vi "FVT.vi"(7 "FrequencyCounter":refnum<visa-resource-name>, 8 "error in":errorcluster, 9 "connection information":path, 10 "System Number":string, 11 "Arduino":refnum<visa-resource-name>) -> (0 "error out":errorcluster, 3 "Arduino out":refnum<visa-resource-name>)   [LabVIEW 2024]
uses:
  <vilib>/addons/database/Connection.llb/DB Tools Open Connec (Path).vi
  Agilent 532XX Series/Public/Configure/Measurement/Configure Measurement (Frequency).vi
  <vilib>/Utility/file.llb/Write Delimited Spreadsheet (string).vi
  <vilib>/addons/database/_DB Variant To Data/Database Variant To Data.xnode
  <vilib>/addons/database/NI_Database_API.lvlib
  Agilent 532XX Series/Agilent 532XX Series.lvlib
panel:
  out "OscVoltage":string
  out "TimeStart":string
  out "StartTime":string
  out "FirstPrint":bool
  out "FirstTime":bool
  out "Path":string
  out "PDF Path":string
  out "Work Order":string
  out "Unit_Number":string
  out "Serial Numbers":string[](array[string])
  in  "System Status":string
  out "Frequency":string
  out "Temperature":string
  out "Nominal Frequency":string
  in  "DC_SN":string
  out "IsSine":bool=TRUE
types:
  T1 = typedef "NI_Database_API.lvlib/Conn ObjectReference.ctl" = refnum<k1>
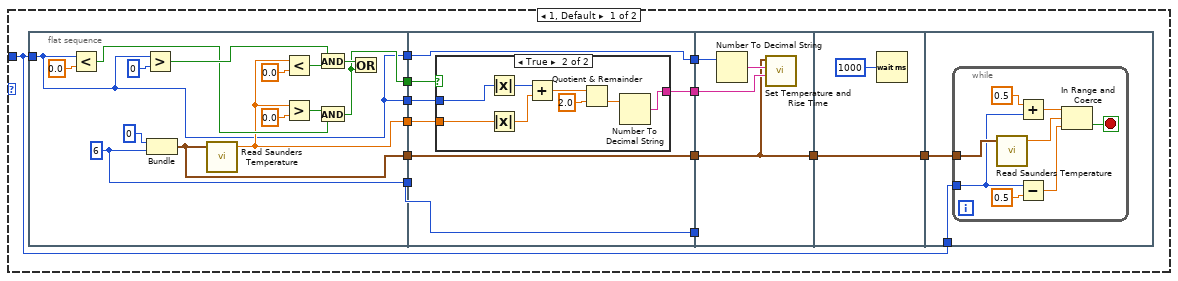
[diagram p2: hidden frame]
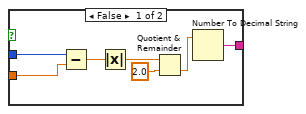
[diagram p3: hidden frame]
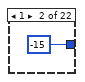
[diagram p4: hidden frame]
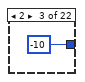
[diagram p5: hidden frame]
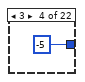
[diagram p6: hidden frame]
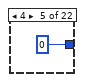
[diagram p7: hidden frame]
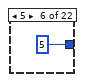
[diagram p8: hidden frame]
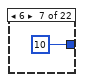
[diagram p9: hidden frame]
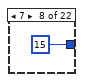
[diagram p10: hidden frame]
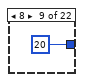
[diagram p11: hidden frame]
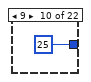
[diagram p12: hidden frame]
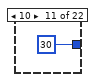
[diagram p13: hidden frame]
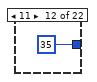
[diagram p14: hidden frame]
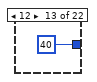
[diagram p15: hidden frame]
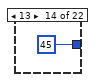
[diagram p16: hidden frame]
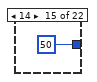
[diagram p17: hidden frame]
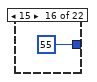
[diagram p18: hidden frame]
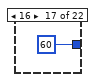
[diagram p19: hidden frame]
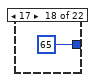
[diagram p20: hidden frame]
diagram:
  n1 = flat-sequence {
    tunnel: "Arduino" -> [w19]
    tunnel: "error in" -> [w18]
    tunnel: [w17] -> w2
    tunnel: [w16] -> w1
    tunnel: [w34] -> w6
    tunnel: [w35] -> w4
    tunnel: w2 -> [w37]
    tunnel: w1 -> [w36]
    tunnel: w6 -> [w733]
    tunnel: [w733] -> w5
    tunnel: w4 -> [w732]
    tunnel: [w732] -> w3
    tunnel: [w773] -> w11
    tunnel: w5 -> [w773]
    tunnel: [w772] -> w9
    tunnel: w3 -> [w772]
    tunnel: [w771] -> w7
    tunnel: w11 -> [w779]
    tunnel: [w779] -> w10
    tunnel: w9 -> [w778]
    tunnel: [w778] -> w8
    tunnel: w7 -> [w777]
    tunnel: w10 -> [w785]
    tunnel: w8 -> [w784]
    tunnel: [w785] -> w13
    tunnel: [w784] -> w12
    frame #0 {
      n2 = Build Array("<48,0>" ("string"), "<50,0>" ("string"), "<52,0>" ("string")) -> (w20:string[])
      n3 = Get Date/Time In Seconds() -> (seconds since 1Jan1904=w29:timestamp)
      n4 = Format Date/Time String(time format string (%c)="%x_%I-%M" ("string"), seconds (now)=w29) -> (date/time string=w28:string)  [unwired: 1 in]
      n5 = call "Arduino Command Builder.vi"("error in"=w18, "Commands"=w20, "Arduino in"=w19) -> ("error out"=w17:errorcluster, "Arduino out"=w16:refnum<visa-resource-name>)  [unwired: 7 in]
      n6 = Search and Replace String(replace all?=TRUE ("replace all? (F)"), input string=w28, search string="/", replace string="-" ("replace string (\"\")")) -> (result string=→"StartTime":string)  [unwired: 4 in, 3 out]
      "FirstTime" <- TRUE ("FirstTime")
      "FirstPrint" <- TRUE ("FirstPrint")
      "Serial Numbers" <- string[] []
    }
    frame #1 {
      n7 = for {
        N: 22 -> [_]
        shift-right: [w40] -> w34
        shift-left: w37 -> [w43]
        shift-right: [w41] -> w35
        shift-left: w36 -> [w42]
        i -> [w39]
        n8 = flat-sequence {
          tunnel: w39 -> [w44]
          tunnel: w43 -> [w156]
          tunnel: w42 -> [w155]
          tunnel: [w154] -> w40
          tunnel: [w153] -> w41
          tunnel: w39 -> [w152]
          frame #0 {
            n9 = case shown="0, Default" w44 {
              tunnel: [-20 -15 -10 -5 0 5 10 15 20 25 30 35 40 45 50 55 60 65 70 75 80 85] -> w45
              frame 0, Default {
              }
              frame 1 {
              }
              frame 2 {
              }
              frame 3 {
              }
              frame 4 {
              }
              frame 5 {
              }
              frame 6 {
              }
              frame 7 {
              }
              frame 8 {
              }
              frame 9 {
              }
              frame 10 {
              }
              frame 11 {
              }
              frame 12 {
              }
              frame 13 {
              }
              frame 14 {
              }
              frame 15 {
              }
              frame 16 {
              }
              frame 17 {
              }
              frame 18 {
              }
              frame 19 {
              }
              frame 20 {
              }
              frame 21 {
              }
            }
            n10 = case shown="0" w44 {
              tunnel: w45 -> [w46 w112]
              frame 1, Default {
                n11 = flat-sequence {
                  tunnel: w46 -> [w59]
                  tunnel: [w59] -> w58
                  tunnel: [w73] -> w57
                  tunnel: [w71] -> w56
                  tunnel: [w61] -> w55
                  tunnel: [w60] -> w54
                  tunnel: [w59] -> w53
                  tunnel: w58 -> [w80]
                  tunnel: [w80] -> w52
                  tunnel: [w74] -> w51
                  tunnel: w57 -> [w79]
                  tunnel: [w79] -> w50
                  tunnel: w56 -> [w78]
                  tunnel: [w78] -> w49
                  tunnel: w55 -> [w77]
                  tunnel: w54 -> [w76]
                  tunnel: w53 -> [w75]
                  tunnel: [w96] -> w48
                  tunnel: w52 -> [w98]
                  tunnel: w51 -> [w97]
                  tunnel: w50 -> [_]
                  tunnel: w49 -> [w96]
                  tunnel: [w100] -> w47
                  tunnel: w48 -> [w100]
                  tunnel: w46 -> [w103]
                  tunnel: w47 -> [w102]
                  frame #0 {
                    w73 = 6
                    n12 = Less?(x=w59, y=0.0) -> (x < y?=w65:bool)
                    n13 = Greater?(x=w59, y=0) -> (0:w68:bool)
                    n14 = Bundle(0, w73) -> (w71:cluster{i32, i32})  [unwired: 1 in]
                    n15 = call "Read Saunders Temperature.vi"("Device"=w71) -> ("Temperature"=w60:dbl)  [unwired: 3 in, 1 out]
                    n16 = Less?(x=w60, y=0.0) -> (x < y?=w67:bool)
                    n17 = Greater?(x=w60, y=0.0) -> (0:w66:bool)
                    n18 = And(x=w68, y=w67) -> (x .and. y?=w64:bool)
                    n19 = And(x=w66, y=w65) -> (x .and. y?=w61:bool)
                    n20 = Or(x=w64, y=w61) -> ()  [unwired: 1 out]
                  }
                  frame #1 {
                    n21 = case shown="True" w77 {
                      tunnel: w76 -> [w86 w94]
                      tunnel: w75 -> [w87 w95]
                      tunnel: [w82 w91] -> w74
                      frame False {
                        n22 = Subtract(x=w87, y=w86) -> (x-y=w85:dbl)
                        n23 = Absolute Value(x=w85) -> (abs(x)=w81:dbl)
                        n24 = Quotient & Remainder(x=w81, y=2.0) -> (floor(x/y)=w83:dbl)  [unwired: 1 out]
                        n25 = Number To Decimal String(number=w83) -> (decimal integer string=w82:string)  [unwired: 1 in]
                      }
                      frame True {
                        n26 = Absolute Value(x=w95) -> (abs(x)=w92:i32)
                        n27 = Absolute Value(x=w94) -> (abs(x)=w93:dbl)
                        n28 = Add(x=w92, y=w93) -> (x+y=w88:dbl)
                        n29 = Quotient & Remainder(x=w88, y=2.0) -> (floor(x/y)=w89:dbl)  [unwired: 1 out]
                        n30 = Number To Decimal String(number=w89) -> (decimal integer string=w91:string)  [unwired: 1 in]
                      }
                    }
                  }
                  frame #2 {
                    n31 = Number To Decimal String(number=w98) -> (decimal integer string=w99:string)  [unwired: 1 in]
                    n32 = call "Set Temperature and Rise Time.vi"("Slew Time String"=w97, "Temperature String"=w99, "Device"=w96) -> ()  [unwired: 3 in, 1 out]
                  }
                  frame #3 {
                    n33 = Wait (ms)(milliseconds to wait=u32 1000) -> ()  [unwired: 1 out]
                  }
                  frame #4 {
                    n34 = while {
                      tunnel: w102 -> [w111]
                      tunnel: w103 -> [w108]
                      stop <- w110 stop-if-true
                      n35 = call "Read Saunders Temperature.vi"("Device"=w111) -> ("Temperature"=w109:dbl)  [unwired: 3 in, 1 out]
                      n36 = Add(x=0.5, y=w108) -> (x+y=w104:dbl)
                      n37 = Subtract(x=w108, y=0.5) -> (x-y=w106:dbl)
                      n38 = In Range and Coerce(upper limit=w104, x=w109, lower limit=w106) -> (In Range?=w110:bool)  [unwired: 1 out]
                    }
                  }
                }
              }
              frame 0 {
                n39 = flat-sequence {
                  tunnel: w112 -> [w117]
                  frame #0 {
                    n40 = Number To Decimal String(number=w117) -> (decimal integer string=w119:string)  [unwired: 1 in]
                    n41 = Bundle(0, 6) -> (w113:cluster{i32, i32})  [unwired: 1 in]
                    n42 = Wait (ms)(milliseconds to wait=u32 1000) -> ()  [unwired: 1 out]
                    n43 = while {
                      tunnel: w113 -> [w127]
                      tunnel: w117 -> [w124]
                      stop <- w126 stop-if-true
                      n44 = call "Read Saunders Temperature.vi"("Device"=w127) -> ("Temperature"=w125:dbl)  [unwired: 3 in, 1 out]
                      n45 = Add(x=0.5, y=w124) -> (x+y=w120:dbl)
                      n46 = Subtract(x=w124, y=0.5) -> (x-y=w122:dbl)
                      n47 = In Range and Coerce(upper limit=w120, x=w125, lower limit=w122) -> (In Range?=w126:bool)  [unwired: 1 out]
                    }
                    n48 = call "Set Temperature and Rise Time.vi"("Slew Time String"="0", "Temperature String"=w119, "Device"=w113) -> ()  [unwired: 3 in, 1 out]
                  }
                  frame #1 {
                    n49 = Wait (ms)(milliseconds to wait=u32 600000) -> ()  [unwired: 1 out]
                  }
                }
              }
            }
          }
          frame #1 {
            n50 = Wait (ms)(milliseconds to wait=u32 60000) -> ()  [unwired: 1 out]
          }
          frame #2 {
            n51 = for {
              N: 32 -> [_]
              shift-right: [w161] -> w154
              shift-left: w156 -> [w163]
              shift-right: [w160] -> w153
              shift-left: w155 -> [w162]
              tunnel: w152 -> [w158]
              i -> [w159]
              n52 = for {
                N: 8 -> [_]
                shift-right: [w172] -> w161
                shift-left: w163 -> [w177]
                shift-right: [w167] -> w160
                shift-left: w162 -> [w176]
                tunnel: w159 -> [w175]
                tunnel: w158 -> [w166]
                i -> [w178]
                n53 = flat-sequence {
                  tunnel: w177 -> [w181]
                  tunnel: w176 -> [w180]
                  tunnel: [w179] -> w171
                  tunnel: [w180] -> w168
                  tunnel: w178 -> [w185]
                  tunnel: w175 -> [w183]
                  tunnel: [w182] -> w174
                  tunnel: [w217] -> w173
                  tunnel: w171 -> [w216]
                  tunnel: [w216] -> w170
                  tunnel: [w215] -> w169
                  tunnel: w168 -> [w215]
                  tunnel: [w184] -> w165
                  tunnel: w174 -> [w270]
                  tunnel: w173 -> [w269]
                  tunnel: [w268] -> w172
                  tunnel: w170 -> [w267]
                  tunnel: w169 -> [w266]
                  tunnel: [w265] -> w167
                  tunnel: w166 -> [w264]
                  tunnel: w165 -> [w263]
                  frame #0 {
                    n54 = call <vilib>:"Clear Errors.vi"("error in (no error)"=w181) -> ("error out"=w179:errorcluster)  [unwired: 5 in, 1 out]
                  }
                  frame #1 {
                    n55 = local write "DC_SN"("" ("DC.SN")) -> ()
                    n56 = local read "System Number"() -> (w203:string)
                    n57 = local read "connection information"() -> (w186:path)
                    n58 = Increment(x=w185) -> (x+1=w202:i32)
                    n59 = Number To Decimal String(number=w202) -> (decimal integer string=w204:string)  [unwired: 1 in]
                    n60 = Concatenate Strings("WHERE System=" ("SQL Query"), w203, " AND Rack=", w204, ";" ("string")) -> (w187:string)
                    n61 = call-poly <vilib>:"DB Tools Open Connection.vi"("connection information"=w186) -> ("error out"=w197:errorcluster, "connection reference"=w198:T1)  [unwired: 7 in]
                    n62 = call <vilib>:"DB Tools Select Data.vi"("condition"=w187, "error in (no error)"=w197, "columns"=string[] ["Position"], "table"="ACTIVE", "connection reference"=w198) -> ("error out"=w194:errorcluster, "data"=w192:variant[][], "connection reference out"=w196:T1)  [unwired: 1 in]
                    n63 = xnode "Database Variant To Data"("database variant"=w192, "error in (no error)"=w194, "type"=string[][] [] ("DC.SN")) -> ("data"=w191:string[][], "error out"=w195:errorcluster)
                    n64 = call <vilib>:"DB Tools Close Connection.vi"("error in (no error)"=w195, "connection reference"=w196) -> ("error out"=w188:errorcluster)  [unwired: 5 in]
                    n65 = Index Array(array=w191, index (row)=0 ("disabled index (row)"), index (col)=0 ("disabled index (col)")) -> (element=w214:string)
                    n66 = Unbundle By Name(w188) -> ("status"=w201:bool)
                    n67 = call <vilib>:"Delimited String to 1D String Array.vi"("delimiter"=",", "delimited string"=w214) -> ("string array"=w211:string[])  [unwired: 9 in]
                    n68 = Not(x=w201) -> (.not. x?=w200:bool)
                    n69 = Index Array(array=w211, index=w183) -> (element=w210:string)
                    n70 = Increment(x=w183) -> (x+1=w217:i32)
                    n71 = Equal?(x="1", y=w210) -> (x = y?=w199:bool)
                    n72 = Increment(x=w185) -> (x+1=w182:i32)
                    n73 = And(x=w199, y=w200) -> (x .and. y?=w184:bool)
                  }
                  frame #2 {
                    n74 = case shown="True" w263 {
                      tunnel: w270 -> [_ w307]
                      tunnel: w269 -> [_ w306]
                      tunnel: [w271 w302] -> w268
                      tunnel: w267 -> [w271 w305]
                      tunnel: w266 -> [w272 w304]
                      tunnel: [w272 w301] -> w265
                      tunnel: w264 -> [_ w294]
                      frame False {
                      }
                      frame True {
                        n75 = flat-sequence {
                          tunnel: w306 -> [w309]
                          tunnel: w307 -> [w308]
                          tunnel: [w308] -> w278
                          tunnel: [w309] -> w277
                          tunnel: [w310] -> w276
                          tunnel: [w505] -> w286
                          tunnel: w278 -> [w509]
                          tunnel: w277 -> [w508]
                          tunnel: w276 -> [w510]
                          tunnel: [w510] -> w275
                          tunnel: [w507] -> w274
                          tunnel: [w506] -> w273
                          tunnel: [w596] -> w302
                          tunnel: w305 -> [w598]
                          tunnel: w304 -> [w599]
                          tunnel: [w597] -> w301
                          tunnel: [w592] -> w295
                          tunnel: [w595] -> w287
                          tunnel: w286 -> [w595]
                          tunnel: [w594] -> w279
                          tunnel: w275 -> [w593]
                          tunnel: w274 -> [w592]
                          tunnel: w273 -> [w594]
                          tunnel: [w609] -> w296
                          tunnel: w295 -> [w609]
                          tunnel: [w608] -> w288
                          tunnel: w287 -> [w608]
                          tunnel: [w607] -> w280
                          tunnel: w279 -> [w607]
                          tunnel: [w620] -> w300
                          tunnel: [w613] -> w297
                          tunnel: w296 -> [w613]
                          tunnel: [w612] -> w289
                          tunnel: w288 -> [w612]
                          tunnel: [w611] -> w281
                          tunnel: w280 -> [w611]
                          tunnel: [w624] -> w303
                          tunnel: [w623] -> w298
                          tunnel: [w622] -> w290
                          tunnel: [w621] -> w282
                          tunnel: w281 -> [w621]
                          tunnel: w289 -> [w622]
                          tunnel: w297 -> [w623]
                          tunnel: w300 -> [w624]
                          tunnel: w303 -> [w626]
                          tunnel: [w630] -> w299
                          tunnel: w298 -> [w630]
                          tunnel: [w629] -> w291
                          tunnel: w290 -> [w629]
                          tunnel: [w628] -> w283
                          tunnel: w282 -> [w628]
                          tunnel: w299 -> [w654]
                          tunnel: [w653] -> w292
                          tunnel: w291 -> [w653]
                          tunnel: [w652] -> w284
                          tunnel: w283 -> [w652]
                          tunnel: w294 -> [w661]
                          tunnel: [w660] -> w293
                          tunnel: w292 -> [w660]
                          tunnel: [w659] -> w285
                          tunnel: w284 -> [w659]
                          tunnel: w293 -> [w722]
                          tunnel: w285 -> [w721]
                          frame #0 {
                            n76 = case shown="2" w308 {
                              tunnel: ["<42,0>" ("string") "<42,1>" ("string") "<42,0>" ("string") "<42,1>" ("string") "<42,0>" ("string") "<42,1>" ("string") "<42,0>" ("string") "<42,1>" ("string")] -> w316
                              tunnel: ["<44,0>" ("string") "<44,0>" ("string") "<44,1>" ("string") "<44,1>" ("string") "<44,0>" ("string") "<44,0>" ("string") "<44,1>" ("string") "<44,1>" ("string")] -> w317
                              tunnel: ["<46,0>" ("string") "<46,0>" ("string") "<46,0>" ("string") "<46,0>" ("string") "<46,1>" ("string") "<46,1>" ("string") "<46,1>" ("string") "<46,1>" ("string")] -> w318
                              frame 1, Default {
                              }
                              frame 2 {
                              }
                              frame 3 {
                              }
                              frame 4 {
                              }
                              frame 5 {
                              }
                              frame 6 {
                              }
                              frame 7 {
                              }
                              frame 8 {
                              }
                            }
                            n77 = case shown="2" w309 {
                              tunnel: ["<32,0>" ("string") "<32,0>" ("string") "<32,0>" ("string") "<32,0>" ("string") "<32,0>" ("string") "<32,0>" ("string") "<32,0>" ("string") "<32,0>" ("string") "<32,0>" ("string") "<32,0>" ("string") "<32,0>" ("string") "<32,0>" ("string") "<32,0>" ("string") "<32,0>" ("string") "<32,0>" ("string") "<32,0>" ("string") "<32,1>" ("string") "<32,1>" ("string") "<32,1>" ("string") "<32,1>" ("string") "<32,1>" ("string") "<32,1>" ("string") "<32,1>" ("string") "<32,1>" ("string") "<32,1>" ("string") "<32,1>" ("string") "<32,1>" ("string") "<32,1>" ("string") "<32,1>" ("string") "<32,1>" ("string") "<32,1>" ("string") "<32,1>" ("string")] -> w315
                              tunnel: ["<30,0>" ("string") "<30,0>" ("string") "<30,0>" ("string") "<30,0>" ("string") "<30,0>" ("string") "<30,0>" ("string") "<30,0>" ("string") "<30,0>" ("string") "<30,1>" ("string") "<30,1>" ("string") "<30,1>" ("string") "<30,1>" ("string") "<30,1>" ("string") "<30,1>" ("string") "<30,1>" ("string") "<30,1>" ("string") "<30,0>" ("string") "<30,0>" ("string") "<30,0>" ("string") "<30,0>" ("string") "<30,0>" ("string") "<30,0>" ("string") "<30,0>" ("string") "<30,0>" ("string") "<30,1>" ("string") "<30,1>" ("string") "<30,1>" ("string") "<30,1>" ("string") "<30,1>" ("string") "<30,1>" ("string") "<30,1>" ("string") "<30,1>" ("string")] -> w314
                              tunnel: ["<28,0>" ("string") "<28,0>" ("string") "<28,0>" ("string") "<28,0>" ("string") "<28,1>" ("string") "<28,1>" ("string") "<28,1>" ("string") "<28,1>" ("string") "<28,0>" ("string") "<28,0>" ("string") "<28,0>" ("string") "<28,0>" ("string") "<28,1>" ("string") "<28,1>" ("string") "<28,1>" ("string") "<28,1>" ("string") "<28,0>" ("string") "<28,0>" ("string") "<28,0>" ("string") "<28,0>" ("string") "<28,1>" ("string") "<28,1>" ("string") "<28,1>" ("string") "<28,1>" ("string") "<28,0>" ("string") "<28,0>" ("string") "<28,0>" ("string") "<28,0>" ("string") "<28,1>" ("string") "<28,1>" ("string") "<28,1>" ("string") "<28,1>" ("string")] -> w313
                              tunnel: ["<26,0>" ("string") "<26,0>" ("string") "<26,1>" ("string") "<26,1>" ("string") "<26,0>" ("string") "<26,0>" ("string") "<26,1>" ("string") "<26,1>" ("string") "<26,0>" ("string") "<26,0>" ("string") "<26,1>" ("string") "<26,1>" ("string") "<26,0>" ("string") "<26,0>" ("string") "<26,1>" ("string") "<26,1>" ("string") "<26,0>" ("string") "<26,0>" ("string") "<26,1>" ("string") "<26,1>" ("string") "<26,0>" ("string") "<26,0>" ("string") "<26,1>" ("string") "<26,1>" ("string") "<26,0>" ("string") "<26,0>" ("string") "<26,1>" ("string") "<26,1>" ("string") "<26,0>" ("string") "<26,0>" ("string") "<26,1>" ("string") "<26,1>" ("string")] -> w312
                              tunnel: ["<24,0>" ("string") "<24,1>" ("string") "<24,0>" ("string") "<24,1>" ("string") "<24,0>" ("string") "<24,1>" ("string") "<24,0>" ("string") "<24,1>" ("string") "<24,0>" ("string") "<24,1>" ("string") "<24,0>" ("string") "<24,1>" ("string") "<24,0>" ("string") "<24,1>" ("string") "<24,0>" ("string") "<24,1>" ("string") "<24,0>" ("string") "<24,1>" ("string") "<24,0>" ("string") "<24,1>" ("string") "<24,0>" ("string") "<24,1>" ("string") "<24,0>" ("string") "<24,1>" ("string") "<24,0>" ("string") "<24,1>" ("string") "<24,0>" ("string") "<24,1>" ("string") "<24,0>" ("string") "<24,1>" ("string") "<24,0>" ("string") "<24,1>" ("string")] -> w311
                              frame 1, Default {
                              }
                              frame 2 {
                              }
                              frame 3 {
                              }
                              frame 4 {
                              }
                              frame 5 {
                              }
                              frame 6 {
                              }
                              frame 7 {
                              }
                              frame 8 {
                              }
                              frame 9 {
                              }
                              frame 10 {
                              }
                              frame 11 {
                              }
                              frame 12 {
                              }
                              frame 13 {
                              }
                              frame 14 {
                              }
                              frame 15 {
                              }
                              frame 16 {
                              }
                              frame 17 {
                              }
                              frame 18 {
                              }
                              frame 19 {
                              }
                              frame 20 {
                              }
                              frame 21 {
                              }
                              frame 22 {
                              }
                              frame 23 {
                              }
                              frame 24 {
                              }
                              frame 25 {
                              }
                              frame 26 {
                              }
                              frame 27 {
                              }
                              frame 28 {
                              }
                              frame 29 {
                              }
                              frame 30 {
                              }
                              frame 31 {
                              }
                              frame 32 {
                              }
                            }
                            n78 = Build Array(w316, w317, w318, w311, w312, w313, w314, w315) -> (w310:string[])
                          }
                          frame #1 {
                            # "Gets the latest TimeStart from this System/Rack/Position meaning it will be associated with the oscillator that is currently in the spot"
                            n79 = local read "connection information"() -> (w514:path)
                            n80 = local read "System Number"() -> (w547:string)
                            n81 = Number To Decimal String(number=w509) -> (decimal integer string=w505:string)  [unwired: 1 in]
                            n82 = Number To Decimal String(number=w508) -> (decimal integer string=w506:string)  [unwired: 1 in]
                            n83 = Concatenate Strings("WHERE SystemNumber=" ("SQL Query"), w547, "AND RackNumber=" ("string"), w505, "AND PositionNumber=" ("string"), w506, "ORDER BY TimeStart DESC" ("string")) -> (w513:string)
                            n84 = call-poly <vilib>:"DB Tools Open Connection.vi"("connection information"=w514) -> ("error out"=w521:errorcluster, "connection reference"=w522:T1)  [unwired: 7 in]
                            n85 = call <vilib>:"DB Tools Select Data.vi"("condition"=w513, "error in (no error)"=w521, "table"="MASTER", "connection reference"=w522) -> ("error out"=w518:errorcluster, "data"=w516:variant[][], "connection reference out"=w520:T1)  [unwired: 2 in]
                            n86 = xnode "Database Variant To Data"("database variant"=w516, "error in (no error)"=w518, "type"=string[][] [] ("DC.SN")) -> ("data"=w512:string[][], "error out"=w519:errorcluster)
                            n87 = call <vilib>:"DB Tools Close Connection.vi"("error in (no error)"=w519, "connection reference"=w520) -> ("error out"=w511:errorcluster)  [unwired: 5 in]
                            n88 = Index Array(array=w512, index (row)=0 ("disabled index (row)")) -> (element=w526:string[])  [unwired: 1 in]
                            n89 = Unbundle By Name(w511) -> ("status"=w532:bool)
                            n90 = Index Array(array=w526, index=9) -> (element=→"OscVoltage":string)
                            n91 = Index Array(array=w526, index=1) -> (element=w525:string)
                            n92 = Index Array(array=w526, index=2) -> (element=w523:string)
                            n93 = Index Array(array=w526, index=7) -> (element=→"TimeStart":string)
                            n94 = Index Array(array=w526, index=8) -> (element=w540:string)
                            n95 = Index Array(array=w526, index=0) -> (element=w539:string)
                            n96 = Index Array(array=w526, index=12) -> (element=w504:string)
                            n97 = Index Array(array=w526, index=10) -> (element=w541:string)
                            n98 = Not(x=w532) -> ()  [unwired: 1 out]
                            n99 = local write "Nominal Frequency"(w540) -> ()
                            n100 = local write "DC_SN"(w539) -> ()
                            n101 = local write "Unit_Number"(w504) -> ()
                            n102 = Concatenate Strings(w525, "-" ("string"), w523) -> (w503:string)
                            n103 = Equal?(x="Sine", y=w541) -> (x = y?=w507:bool)
                            n104 = local write "Work Order"(w503) -> ()
                          }
                          frame #2 {
                            n105 = case shown="True" w592 {
                              tunnel: w599 -> [w601 w606]
                              tunnel: w598 -> [w600 w605]
                              tunnel: [w601 w604] -> w597
                              tunnel: [w600 w603] -> w596
                              tunnel: w593 -> [_ w602]
                              frame False {
                              }
                              frame True {
                                n106 = call "Arduino Command Builder.vi"("error in"=w605, "Commands"=w602, "Arduino in"=w606) -> ("error out"=w603:errorcluster, "Arduino out"=w604:refnum<visa-resource-name>)  [unwired: 7 in]
                              }
                            }
                          }
                          frame #3 {
                            n107 = Wait (ms)(milliseconds to wait=u32 1000 ("millisecond multiple")) -> ()  [unwired: 1 out]
                          }
                          frame #4 {
                            # "Records the current temperature"
                            n108 = Bundle(0, 6) -> (w619:cluster{i32, i32})  [unwired: 1 in]
                            n109 = call "Read Saunders Temperature.vi"("Device"=w619) -> ("error out 2"=w620:errorcluster, "Temperature"=w617:dbl)  [unwired: 3 in]
                            n110 = Format Into String(format string="%.2f" ("Format String"), w617) -> (resulting string=→"Temperature":string)  [unwired: 2 in, 1 out]
                          }
                          frame #5 {
                            # "This checks if the wave is sine and changes the settings based on the waveform type"
                            n111 = Wait (ms)(milliseconds to wait=u32 500 ("millisecond multiple")) -> ()  [unwired: 1 out]
                          }
                          frame #6 {
                            n112 = for {
                              N: 5 -> [_]
                              tunnel: w626 -> [w632]
                              stop <- w635 continue-if-true
                              w639 = 1 items=["Channel 1"=1, "Channel 2"=2, "Channel 3"=3] ("Channel (1:Channel 1)")
                              n113 = local read "FrequencyCounter"() -> (w646:refnum<visa-resource-name>)
                              n114 = call "Initialize.vi"("error in (no error)"=w632, "VISA resource name"=w646) -> ("error out"=w641:errorcluster, "VISA resource name out"=w640:refnum<visa-resource-name>)  [unwired: 8 in]
                              n115 = call "Configure Frequency Gate.vi"("error in (no error)"=w641, "Time Resolution (0.1 s)"=0.1 ("number"), "VISA resource name"=w640) -> ("error out"=w650:errorcluster, "VISA resource name out"=w647:refnum<visa-resource-name>)  [unwired: 7 in]
                              n116 = call-poly "Configure Measurement.vi"("error in (no error)"=w650, "Channel (1:Channel 1)"=w639, "VISA resource name"=w647) -> ("error out"=w649:errorcluster, "VISA resource name out"=w648:refnum<visa-resource-name>)  [unwired: 2 in, 5 out]
                              n117 = call "Read Measurement (Single).vi"("error in (no error)"=w649, "VISA resource name"=w648) -> ("error out"=w643:errorcluster, "Measurement"=w644:dbl, "VISA resource name out"=w642:refnum<visa-resource-name>)  [unwired: 7 in]
                              n118 = call "Close.vi"("error in (no error)"=w643, "VISA resource name"=w642) -> ("error out"=w645:errorcluster)  [unwired: 9 in]
                              n119 = In Range and Coerce(upper limit=5000000000.0, x=w644, lower limit=0.0) -> (coerced(x)=w633:dbl)  [unwired: 1 out]
                              n120 = Unbundle By Name(w645) -> ("status"=w635:bool)
                              n121 = Format Into String(format string="%.6f", w633) -> (resulting string=→"Frequency":string)  [unwired: 2 in, 1 out]
                              n122 = case shown="False" w635 {
                                frame False {
                                }
                                frame True {
                                n123 = local read "FrequencyCounter"() -> (w651:refnum<visa-resource-name>)
                                n124 = VISA Clear(VISA resource name=w651) -> ()  [unwired: 1 in, 2 out]
                                }
                              }
                            }
                          }
                          frame #7 {
                            n125 = case shown="True" w654 {
                              frame False {
                              }
                              frame True {
                                n126 = local read "connection information"() -> (w655:path)
                                n127 = local read "Temperature"() -> (w657:string)
                                n128 = local read "Frequency"() -> (w656:string)
                                n129 = local read "DC_SN"() -> (w658:string)
                                n130 = call "Update DatabaseF.vi"("Frequency"=w656, "connection information"=w655, "Temperature"=w657, "DC_SN"=w658) -> ()  [unwired: 1 in]
                              }
                            }
                          }
                          frame #8 {
                            n131 = case shown="0" w661 {
                              frame 0 {
                                n132 = flat-sequence {
                                tunnel: [w683] -> w662
                                tunnel: w662 -> [w703]
                                frame #0 {
                                n133 = local read "FirstTime"() -> (w663:bool)
                                n134 = case shown="False" w663 {
                                frame False {
                                }
                                frame True {
                                w666 = "-" ("string")
                                n135 = local write "FirstTime"(FALSE ("FirstTime")) -> ()
                                n136 = Get Date/Time In Seconds() -> (seconds since 1Jan1904=w677:timestamp)
                                n137 = Format Date/Time String(time format string (%c)="%x_%I-%M" ("string"), seconds (now)=w677) -> (date/time string=w676:string)  [unwired: 1 in]
                                n138 = local read "Unit_Number"() -> (w673:string)
                                n139 = local read "Work Order"() -> (w674:string)
                                n140 = Search and Replace String(replace all?=TRUE ("replace all? (F)"), input string=w676, search string="/", replace string="-" ("replace string (\"\")")) -> (result string=w675:string)  [unwired: 4 in, 3 out]
                                n141 = Concatenate Strings("\\\\Bti-dc1\\ATE-Archive\\NewDataArchive\\_FvT\\" ("string"), "FVT-" ("string"), w674, w666, w673, w666, w675) -> (w680:string)
                                "Path" <- w680
                                n142 = String To Path(string=w680) -> (path=w679:path)
                                n143 = call <vilib>:"Check if File or Folder Exists.vi"("path"=w679) -> ("file or folder exists?"=w678:bool, "dup path"=w665:path)  [unwired: 8 in, 1 out]
                                n144 = case shown="False" w678 {
                                tunnel: w665 -> [w681 _]
                                frame False {
                                n145 = Create Folder(path (use dialog)=w681) -> ()  [unwired: 2 in, 3 out]
                                }
                                frame True {
                                }
                                }
                                }
                                }
                                }
                                frame #1 {
                                n146 = local read "DC_SN"() -> (w683:string)
                                n147 = local read "Path"() -> (w682:string)
                                n148 = Concatenate Strings(w682, "\\" ("string"), w683, ".csv" ("string")) -> (w701:string)
                                n149 = String To Path(string=w701) -> (path=w702:path)
                                n150 = Build Array("Unit_Number" ("string"), "Serial_Number" ("element"), "Date_Code" ("element"), "Work_Order" ("element"), "Test_System" ("element"), "Position" ("element"), "Fixture_SN" ("element"), "Run_FileName" ("element"), "Frequency" ("element"), "Temperature" ("element"), "Time_stamp" ("element"), "Run_ID" ("element")) -> (w700:string[])
                                n151 = call-poly <vilib>:"Write Delimited Spreadsheet.vi"("file path (dialog if empty)"=w702, "1D data"=w700, "append to file? (new file:F)"=FALSE, "delimiter (\\t)"="," ("delimiter (\\t)")) -> ()  [unwired: 10 in, 2 out]
                                }
                                frame #2 {
                                n152 = local read "Serial Numbers"() -> (w704:string[])
                                n153 = Insert Into Array(array=w704, new element=w703) -> (w705:string[])  [unwired: 1 in]
                                n154 = local write "Serial Numbers"(w705) -> ()
                                }
                                }
                              }
                              frame 1, Default {
                              }
                            }
                          }
                          frame #9 {
                            n155 = Get Date/Time In Seconds() -> (seconds since 1Jan1904=w730:timestamp)
                            n156 = local read "System Number"() -> (w727:string)
                            n157 = Concatenate Strings(w722, "-" ("string"), w721) -> (w720:string)
                            n158 = local read "Unit_Number"() -> (w726:string)
                            n159 = local read "Temperature"() -> (w707:string)
                            n160 = local read "Work Order"() -> (w729:string)
                            n161 = local read "Frequency"() -> (w706:string)
                            n162 = Format Date/Time String(time format string (%c)="%c", seconds (now)=w730) -> (date/time string=w725:string)  [unwired: 1 in]
                            n163 = local read "DC_SN"() -> (w711:string)
                            n164 = local read "Path"() -> (w710:string)
                            n165 = local read "DC_SN"() -> (w724:string)
                            n166 = Concatenate Strings(w710, "\\" ("string"), w711, ".csv" ("string")) -> (w709:string)
                            n167 = String To Path(string=w709) -> (path=w708:path)
                            n168 = Build Array(w726, w724, w724, w729, w727, w720, "" ("element"), "NONE" ("element"), w706, w707, w725, "1313" ("element")) -> (w728:string[])
                            n169 = call-poly <vilib>:"Write Delimited Spreadsheet.vi"("file path (dialog if empty)"=w708, "1D data"=w728, "append to file? (new file:F)"=TRUE, "delimiter (\\t)"="," ("delimiter (\\t)")) -> ()  [unwired: 10 in, 2 out]
                          }
                        }
                      }
                    }
                  }
                }
              }
            }
          }
        }
      }
    }
    frame #2 {
      n170 = local read "Serial Numbers"() -> (w731:string[])
      n171 = for {
        tunnel: w731 -> [w734] mode=indexing
        n172 = flat-sequence {
          tunnel: [w742] -> w735
          tunnel: w734 -> [w742]
          tunnel: w735 -> [w757]
          frame #0 {
            n173 = Wait (ms)(milliseconds to wait=u32 1000) -> ()  [unwired: 1 out]
            n174 = local write "System Status"("Converting Files to Winplot PDFs") -> ()
          }
          frame #1 {
            w743 = "-" ("string")
            n175 = local read "Unit_Number"() -> (w747:string)
            n176 = local read "Work Order"() -> (w748:string)
            n177 = local read "StartTime"() -> (w738:string)
            n178 = local read "FirstPrint"() -> (w739:bool)
            n179 = Concatenate Strings("\\\\Bti-dc1\\ate\\Winplots\\" ("string"), "FVT-" ("string"), w748, w743, w747, w743, w738) -> (w744:string)
            n180 = case shown="True" w739 {
              tunnel: w744 -> [_ w750]
              frame False {
              }
              frame True {
                n181 = String To Path(string=w750) -> (path=w751:path)
                n182 = local write "FirstPrint"(FALSE ("FirstPrint")) -> ()
                n183 = call <vilib>:"Check if File or Folder Exists.vi"("path"=w751) -> ("file or folder exists?"=w752:bool, "dup path"=w753:path)  [unwired: 8 in, 1 out]
                n184 = case shown="False" w752 {
                  tunnel: w753 -> [w754 _]
                  frame False {
                    n185 = Create Folder(path (use dialog)=w754) -> ()  [unwired: 2 in, 3 out]
                  }
                  frame True {
                  }
                }
              }
            }
            n186 = Concatenate Strings(w744, "\\" ("string"), w742) -> (w741:string)
            n187 = local write "PDF Path"(w741) -> ()
          }
          frame #2 {
            n188 = local read "Path"() -> (w759:string)
            n189 = Concatenate Strings(w759, "\\" ("string"), w757, ".csv" ("string")) -> (w755:string)
            n190 = local read "PDF Path"() -> (w768:string)
            n191 = Open Python Session(python version="3.12" ("Python version")) -> (session out=w767:refnum<k35>, error out=w766:errorcluster)  [unwired: 2 in]
            n192 = node ("Python Node")(w767, path "C:/Users/golden_apple_1/Desktop/Testing/convert.py" ("module path"), "load_data" ("function name"), w766, string[] [], w755, w768) -> (w765:refnum<k35>, w764:errorcluster)  [unwired: 3 in, 2 out]
            n193 = Close Python Session(session in=w765, error in=w764) -> ()  [unwired: 1 out]
          }
          frame #3 {
            n194 = Wait (ms)(milliseconds to wait=u32 10000) -> ()  [unwired: 1 out]
          }
        }
      }
    }
    frame #3 {
      n195 = Bundle(0, 6) -> (w771:cluster{i32, i32})  [unwired: 1 in]
      n196 = call "Set Temperature and Rise Time.vi"("Slew Time String"="0", "Temperature String"="25", "Device"=w771) -> ()  [unwired: 3 in, 1 out]
    }
    frame #4 {
      # "Brings temp back down to normal range"
      n197 = while {
        tunnel: w777 -> [w783]
        stop <- w780 stop-if-true
        n198 = call "Read Saunders Temperature.vi"("Device"=w783) -> ("Temperature"=w781:dbl)  [unwired: 3 in, 1 out]
        n199 = Less?(x=w781, y=50.0 ("lower limit")) -> (x < y?=w780:bool)
      }
    }
    frame #5 {
      # "Turns off Saunders Temp Machine"
      n200 = Bundle(0, 6) -> (w786:cluster{i32, i32})  [unwired: 1 in]
      n201 = call "Set Temperature and Rise Time.vi"("Temperature String"="o", "Device"=w786) -> ()  [unwired: 4 in, 1 out]
    }
  }
  "error out" <- w13
  "Arduino out" <- w12
